vi "Withdraw.vi"(8 "error in (no error)":errorcluster, 10 "Amount":dbl, 11 "IWithdrawable in":refnum<class "IWithdrawable.lvclass">) -> (0 "error out":errorcluster, 1 "Success?":bool, 2 "Balance":dbl, 3 "IWithdrawable out":refnum<class "IWithdrawable.lvclass">)   [LabVIEW 2020, in "IWithdrawable.lvclass"]
uses:
  IWithdrawable.lvclass
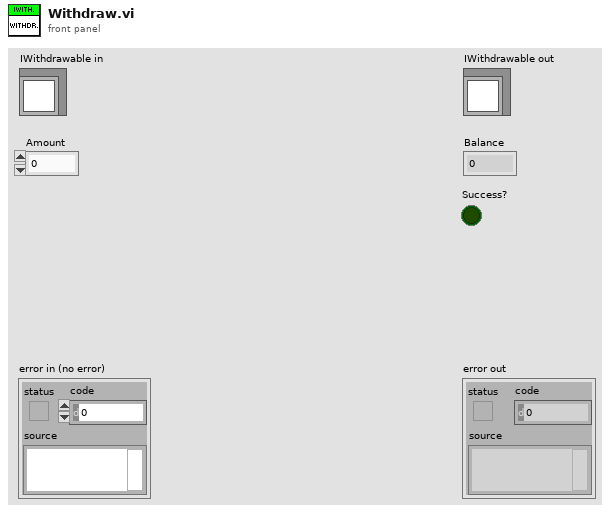
[diagram p1: front panel]
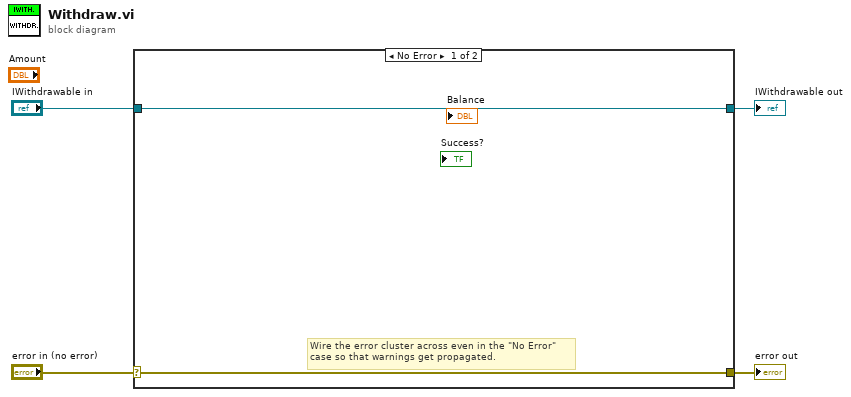
[diagram p0: block diagram]
diagram:
  n1 = case shown="No Error" "error in (no error)" {
    selector: "error in (no error)" -> [w5 w8]
    tunnel: [w5 w8] -> w3
    tunnel: [w6 w7] -> w1
    tunnel: "IWithdrawable in" -> [w6 w7]
    frame No Error {
      # "Wire the error cluster across even in the \"No Error\"\ncase so that warnings get propagated."
    }
    frame Error {
    }
  }
  "error out" <- w3
  "IWithdrawable out" <- w1
